vi "RemoveEmptyRows.vi"(8 "Error In":errorcluster, 11 "Input array with empty rows":string[][](array[string])) -> (0 "Error Out":errorcluster, 3 "array w/ subset deleted":string[][](array[string]))   [LabVIEW 2014]
uses:
  Controls/ColumnHeaders1.ctl
  <userlib>/_RADE/MTA-lib/array/array.llb/Search 1D Array (String)__ogtk.vi
  <userlib>/_RADE/MTA-lib/array/array.llb/Delete Elements from 2D Array (String)__ogtk.vi
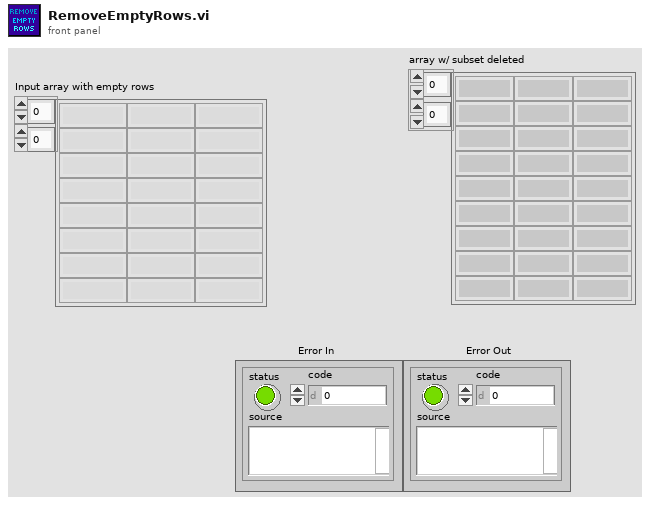
[diagram p1: front panel]
types:
  T1 = typedef "ColumnHeaders1.ctl" = enum16{"Store", "Display", "Method", "Property", "Unit", "URL", "IP Address", "Data Block", "Address", "Data Type"}
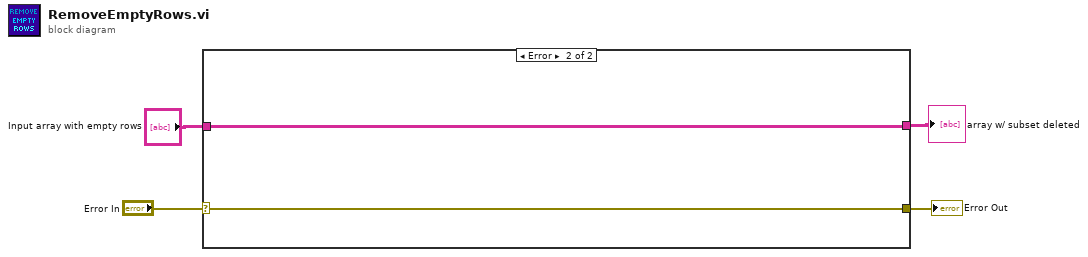
[diagram p0: block diagram]
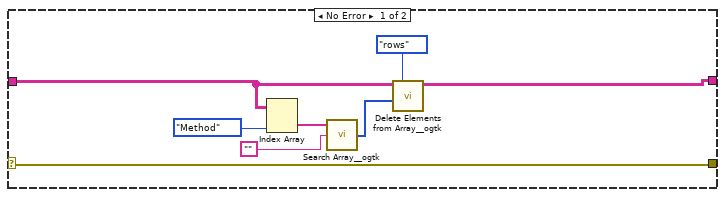
[diagram p2: hidden frame]
diagram:
  n1 = case shown="Error" "Error In" {
    selector: "Error In" -> [w5 w13]
    tunnel: [w7 w14] -> w4
    tunnel: "Input array with empty rows" -> [w6 w14]
    tunnel: [w5 w13] -> w1
    frame No Error {
      n2 = Index Array(array=w6, index (col)=ColumnHeaders1."Method" ("ColumnHeaders")) -> (element=w11:string[])  [unwired: 1 in]
      n3 = call-poly <userlib>:"Search Array__ogtk.vi"("Array"=w11, "Element Data"="") -> ("Indices of Elements"=w10:i32[])  [unwired: 7 in]
      n4 = call-poly <userlib>:"Delete Elements from Array__ogtk.vi"("delete (rows or columns)"=enum16{"rows", "columns"}."rows", "indices"=w10, "array"=w6) -> ("array w/ subset deleted"=w7:string[][])  [unwired: 7 in, 1 out]
    }
    frame Error {
    }
  }
  "array w/ subset deleted" <- w4
  "Error Out" <- w1
